vi "Array Set Element At (Dimension).vi"(8 "error in (no error)":errorcluster, 9 "Element":refnum<data-value>, 10 "Index":i32[](array[numeric]), 11 "Array DVR in":refnum<data-value>) -> (0 "error out":errorcluster, 3 "Array DVR out":refnum<data-value>)   [LabVIEW 2012, in "MDSplus.lvlib"]
uses:
  <vilib>/MDSplus/Library/MDSplus.lvlib
  <vilib>/MDSplus/Classes/Data_Class/Array_Class/Array.lvclass
  <vilib>/MDSplus/Classes/Data_Class/Data.lvclass
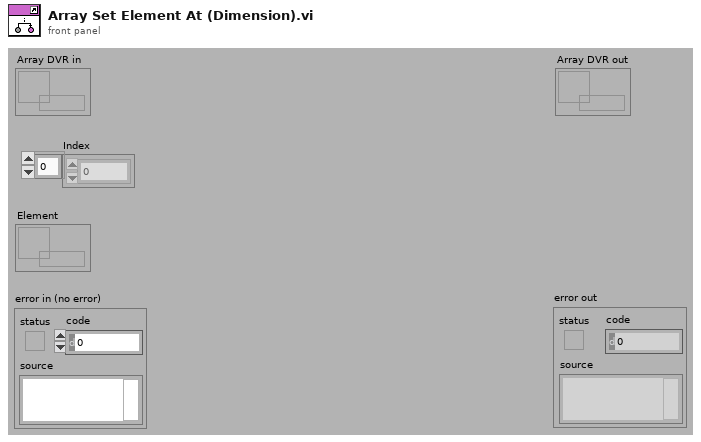
[diagram p1: front panel]
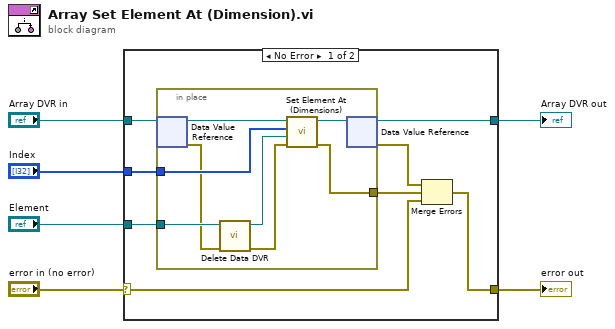
[diagram p0: block diagram]
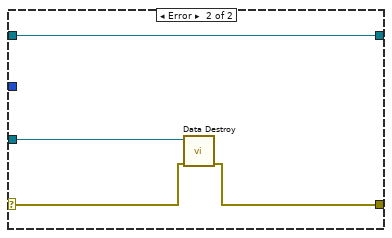
[diagram p2: hidden frame]
diagram:
  n1 = case shown="No Error" "error in (no error)" {
    selector: "error in (no error)" -> [w12 w24]
    tunnel: "Array DVR in" -> [w14 w26]
    tunnel: [w11 w23] -> w6
    tunnel: [w10 w26] -> w3
    tunnel: "Index" -> [w9 _]
    tunnel: "Element" -> [w7 w25]
    frame No Error {
      n2 = in-place {
        in-place-border: [w19] -> w13
        in-place-border: w9 -> [w20]
        in-place-border: w7 -> [w18]
        n3 = in-place-dvr #1(w14) -> (w22:refnum<class "Array.lvclass">, w17:errorcluster)
        n4 = call <vilib>:"Delete Data DVR.vi"("error in (no error)"=w17, "Data DVR in"=w18) -> ("error out"=w15:errorcluster, "Data out"=w16:refnum<class "Data.lvclass">)  [unwired: 8 in]
        n5 = call-dynamic "Set Element At (Dimensions).vi"("error in (no error)"=w15, "Element"=w16, "Index"=w20, "Array in"=w22) -> ("error out"=w19:errorcluster, "Array out"=w21:refnum<class "Array.lvclass">)  [unwired: 6 in]
        n6 = in-place-dvr #1(w21) -> (w10:refnum<data-value>, w8:errorcluster)
      }
      n7 = Merge Errors(w8, w13, w12) -> (w11:errorcluster)
    }
    frame Error {
      n8 = call <vilib>:"Data Destroy.vi"("error in (no error)"=w24, "Data DVR in"=w25) -> ("error out"=w23:errorcluster)  [unwired: 9 in]
    }
  }
  "error out" <- w6
  "Array DVR out" <- w3
